vi "Custom Constant Dialog.vi"(8 "error in":errorcluster, 11 "Selection":T1) -> (0 "error out":errorcluster, 2 "Cancel Out":bool, 3 "New Constant VI name":string)   [LabVIEW 2020, in "ConstantErrorsMaker.lvlib"]
uses:
  ConstantErrorsMaker.lvlib
  MulticolumListbox.ctl
  Selection Type--enum.ctl
  Selection Info--cluster.ctl
panel:
  in  "Project Results":T3 caption="Project Results Table"
  in  "New Constant VI name (do not add --constant.vi)":string
  in  "Continue":bool
  in  "Cancel":bool
  # "TIP: Doble click to open --error.vi Block Diagram"
  # "Constant VIs help manage fixed values efficiently. They work like regular constants but allow centralized editing.\n\nKey Benefits:\n\nSingle Point of Editing: Update the value in one place, and changes apply everywhere.\n\nBetter Maintainability: Clear, modular code makes it easy to find and modify values.\n\nFewer Errors: Reduces typos and inconsistencies across your application."
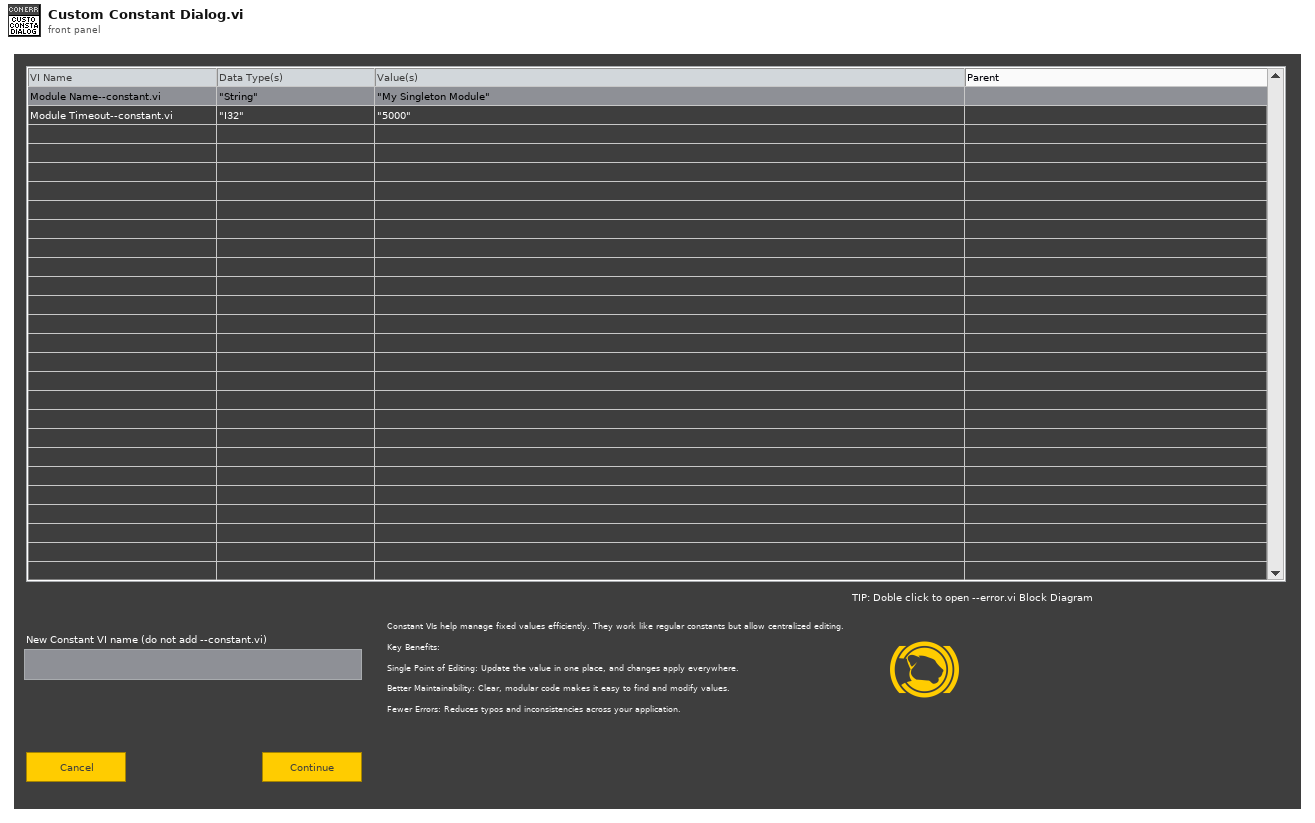
[diagram p1: front panel]
types:
  T1 = typedef "ConstantErrorsMaker.lvlib/Selection Info--cluster.ctl" = cluster{"Name":string, "Library Ref":refnum<vi>, "Application Instance":refnum<vi>, "Selection Owning Folder":path, "Selection Type":T2, "Project Reference":refnum<vi>, "LVClassLibrary Refnum":refnum<vi>}
  T2 = typedef "ConstantErrorsMaker.lvlib/Selection Type--enum.ctl" = enum16{"Project", "Library", "Class"}
  T3 = typedef "ConstantErrorsMaker.lvlib/MulticolumListbox.ctl" = i32
  T4 = typedef "ConstantErrorsMaker.lvlib/Constant Info--cluster.ctl" = cluster{"VI Name":string, "Data Type(s)":string, "Value(s)":string, "Parent":string}
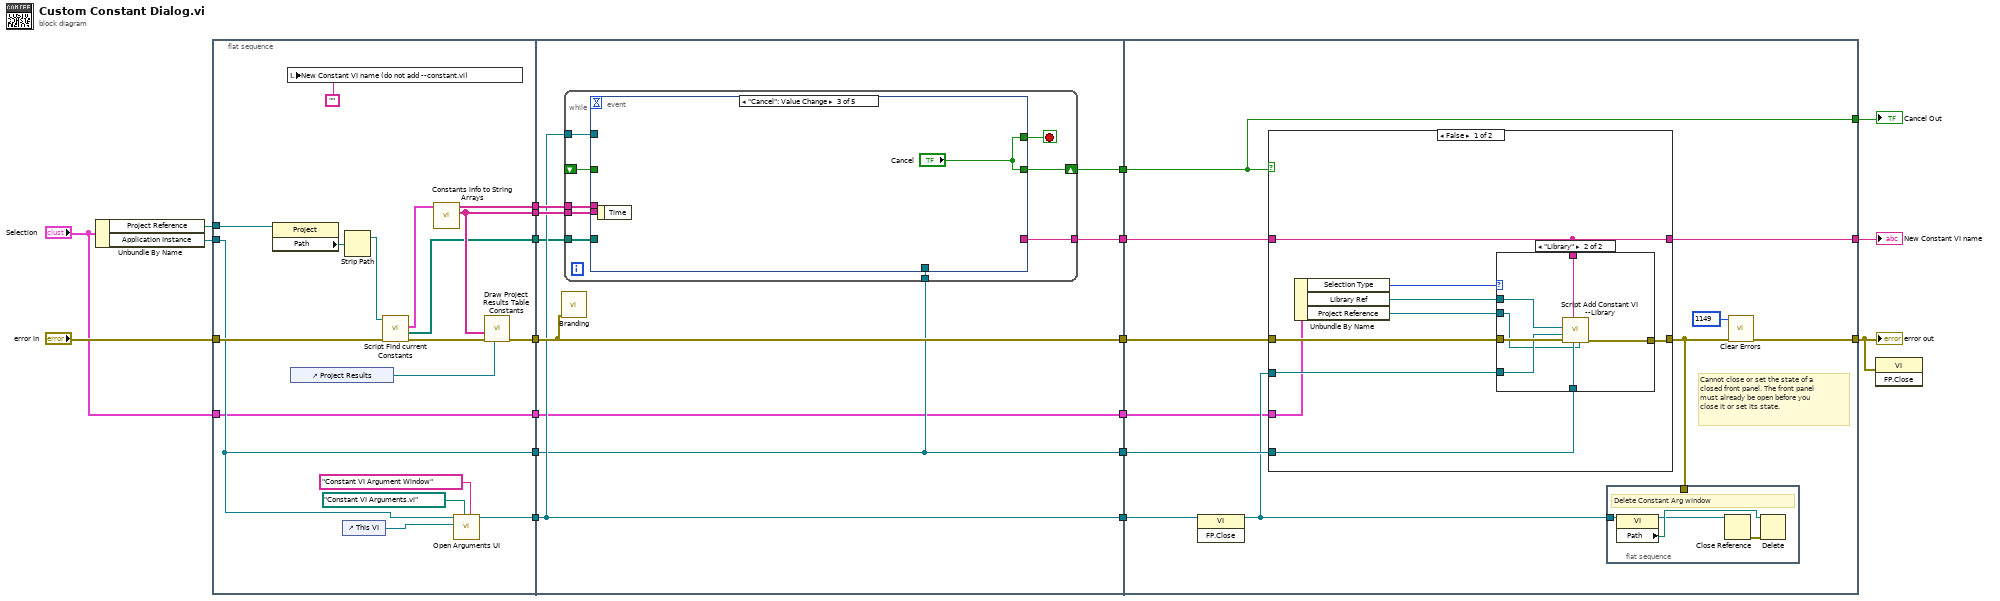
[diagram p0: block diagram]
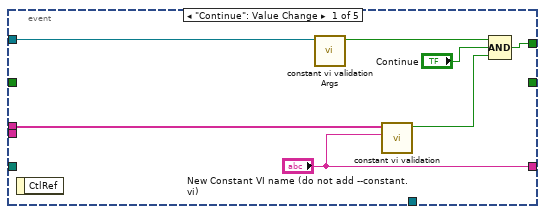
[diagram p2: hidden frame]
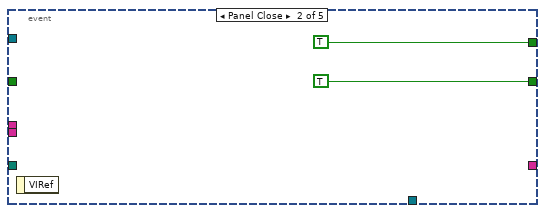
[diagram p3: hidden frame]
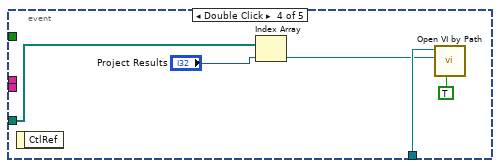
[diagram p4: hidden frame]
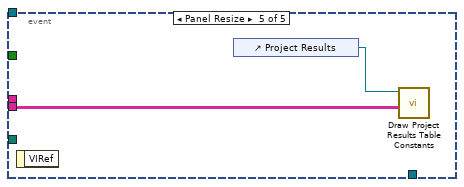
[diagram p5: hidden frame]
diagram:
  n1 = Unbundle By Name("Selection") -> ("Project Reference"=w5:refnum<vi>, "Application Instance"=w4:refnum<vi>)
  n2 = flat-sequence {
    tunnel: [w34] -> w14
    tunnel: [w22] -> w13
    tunnel: [w29] -> w8
    tunnel: [w28] -> w7
    tunnel: [w37] -> w19
    tunnel: "error in" -> [w36]
    tunnel: [w26] -> w6
    tunnel: w5 -> [w25]
    tunnel: w4 -> [w22]
    tunnel: [w21] -> w3
    tunnel: "Selection" -> [w21]
    tunnel: [w47] -> w20
    tunnel: [w45] -> w16
    tunnel: [w42] -> w15
    tunnel: w14 -> [w42]
    tunnel: w13 -> [w40]
    tunnel: [w40] -> w12
    tunnel: [w46] -> w11
    tunnel: w8 -> [w44]
    tunnel: w7 -> [w43]
    tunnel: w19 -> [w47]
    tunnel: w6 -> [w41]
    tunnel: w3 -> [w39]
    tunnel: [w39] -> w1
    tunnel: [w84] -> w17
    tunnel: w20 -> [w82]
    tunnel: w16 -> [w75]
    tunnel: w15 -> [w81]
    tunnel: w12 -> [w80]
    tunnel: w11 -> [w79]
    tunnel: [w76] -> w10
    tunnel: [w75] -> w9
    tunnel: w1 -> [w74]
    frame #0 {
      n3 = property class="Project"(reference=w25) -> ("Path"=w24:path)  [unwired: 1 in, 2 out]
      n4 = local write "New Constant VI name (do not add --constant.vi)"("") -> ()
      n5 = control-ref of="Project Results"() -> (w27:refnum<vi>)
      n6 = control-ref of="This VI"() -> (w35:refnum<vi>)
      n7 = Strip Path(path=w24) -> (stripped path=w23:path)  [unwired: 1 out]
      n8 = call "Script Find current Constants.vi"("error in"=w36, "Selction Owning Folder"=w23) -> ("error out"=w38:errorcluster, "All Constant VIS"=w26:path[], "Constants Info"=w30:T4[])  [unwired: 7 in]
      n9 = call "Constants info to String Arrays.vi"("Constants Info"=w30) -> ("Constant Info Results Str"=w29:string[][], "VI Names"=w28:string[])  [unwired: 9 in]
      n10 = call "Open Arguments UI.vi"("Title"="Constant VI Argument Window", "Path"=path "Constant VI Arguments.vi", "Calling VI Ref"=w35, "App Instance"=w22) -> ("Error Arguments Window Ref"=w34:refnum<vi>)  [unwired: 6 in, 1 out]
      n11 = call "Draw Project Results Table Constants.vi"("error in"=w38, "Constant Results"=w29, "Project Results Ref"=w27) -> ("error out"=w37:errorcluster)  [unwired: 8 in]
    }
    frame #1 {
      n12 = call "Branding.vi"("error in"=w47) -> ()  [unwired: 11 in]
      n13 = while {
        tunnel: w42 -> [w54]
        shift-right: [w55] -> w45
        shift-left: _ -> [w53]
        tunnel: [w52] -> w46
        tunnel: w44 -> [w51]
        tunnel: w43 -> [w50]
        tunnel: w41 -> [w49]
        tunnel: w40 -> [w48]
        stop <- w56 stop-if-true
        n14 = event shown="[2] \"Cancel\": Value Change" {
          selector: _ -> [_ _ _ _ _]
          dyn-events: _ -> [_ _ _ _ _]
          timeout: _ -> [_ _ _ _ _]
          tunnel: [w63 TRUE ("Cancel") "Cancel" _ _] -> w56
          tunnel: [_ TRUE ("Cancel") "Cancel" _ _] -> w55
          tunnel: w54 -> [w58 _ _ _ _]
          tunnel: w53 -> [_ _ _ _ _]
          tunnel: ["New Constant VI name (do not add --constant.vi)" _ _ _ _] -> w52
          tunnel: w50 -> [w57 _ _ _ _]
          tunnel: w51 -> [_ _ _ _ w73]
          tunnel: w49 -> [_ _ _ w70 _]
          tunnel: w48 -> [_ _ _ w71 _]
          event "Continue": Value Change {
            n15 = event-data() -> ()  [unwired: 1 in, 1 out]
            n16 = call "constant vi validation Args.vi"("Constant Argument Window"=w58) -> ("Proceed with Scripting"=w61:bool)  [unwired: 10 in]
            n17 = call "constant vi validation.vi"("New Constant vi name"="New Constant VI name (do not add --constant.vi)", "Constant VI List"=w57) -> ("Proceed with Scripting"=w60:bool)  [unwired: 9 in]
            n18 = Compound Arithmetic op=AND(w61, "Continue", w60) -> (w63:bool)
          }
          event Panel Close {
            n19 = event-data() -> ()  [unwired: 1 in, 1 out]
          }
          event "Cancel": Value Change {
            n20 = event-data() -> ()  [unwired: 1 in, 1 out]
          }
          event Double Click {
            n21 = event-data() -> ()  [unwired: 1 in, 1 out]
            n22 = Index Array(array=w70, index="Project Results") -> (element=w68:path)
            n23 = call "Open VI by Path.vi"("Block Diagram?"=TRUE, "VI Path"=w68, "Application in"=w71) -> ()  [unwired: 8 in, 1 out]
          }
          event Panel Resize {
            n24 = event-data() -> ()  [unwired: 1 in, 1 out]
            n25 = control-ref of="Project Results"() -> (w72:refnum<vi>)
            n26 = call "Draw Project Results Table Constants.vi"("Constant Results"=w73, "Project Results Ref"=w72) -> ()  [unwired: 9 in, 1 out]
          }
        }
      }
    }
    frame #2 {
      # "Cannot close or set the state of a closed front panel. The front panel must already be open before you close it or set its state."
      n27 = invoke class="VI" method="FP.Close"(reference=w81) -> (reference out=w77:refnum<vi>)  [unwired: 2 in, 2 out]
      n28 = case shown="False" w75 {
        tunnel: [w96 w107] -> w83
        tunnel: w82 -> [w97 w107]
        tunnel: w77 -> [w95 _]
        tunnel: w80 -> [w94 _]
        tunnel: w79 -> [w93 w106]
        tunnel: [w93 w106] -> w76
        tunnel: w74 -> [w92 _]
        frame False {
          n29 = Unbundle By Name(w92) -> ("Selection Type"=w91:T2, "Library Ref"=w90:refnum<vi>, "Project Reference"=w89:refnum<vi>)
          n30 = case shown="\"Library\"" w91 {
            tunnel: w97 -> [w98 w105]
            tunnel: [w98 w104] -> w96
            tunnel: w95 -> [_ w103]
            tunnel: w94 -> [_ w102]
            tunnel: w93 -> [_ w101]
            tunnel: w90 -> [_ w100]
            tunnel: w89 -> [_ w99]
            frame "Project", Default {
            }
            frame "Library" {
              n31 = call "Script Add Constant VI --Library.vi"("Project Ref"=w99, "App Ref"=w102, "Constant VI Name"=w101, "error in"=w105, "Constant VI Args"=w103, "Library Reference"=w100) -> ("error out"=w104:errorcluster)  [unwired: 4 in, 1 out]
            }
          }
        }
        frame True {
        }
      }
      n32 = flat-sequence {
        tunnel: w77 -> [w87]
        tunnel: w83 -> [_]
        frame #0 {
          # "Delete Constant Arg window"
          n33 = property class="VI"(reference=w87) -> (reference out=w85:refnum<vi>, "Path"=w86:path)  [unwired: 1 in, 1 out]
          n34 = Close Reference(reference=w85) -> (error out=w88:errorcluster)  [unwired: 1 in]
          n35 = Delete(path (use dialog)=w86, error in=w88) -> ()  [unwired: 3 in, 3 out]
        }
      }
      n36 = call <vilib>:"Clear Errors.vi"("error in (no error)"=w83, "specific error code to clear (0: all)"=1149) -> ("error out"=w84:errorcluster)  [unwired: 4 in, 1 out]
    }
  }
  n37 = invoke class="VI" method="FP.Close"(error in=w17) -> ()  [unwired: 2 in, 3 out]
  "error out" <- w17
  "New Constant VI name" <- w10
  "Cancel Out" <- w9
